vi "average_v2.vi"(4 "Numeric 8":fxp<+/-,24,1>, 5 "Numeric":fxp<+/-,24,1>, 6 "Numeric 7":fxp<+/-,24,1>, 7 "Numeric 2":fxp<+/-,24,1>, 8 "Numeric 6":fxp<+/-,24,1>, 9 "Numeric 5":fxp<+/-,24,1>, 10 "Numeric 4":fxp<+/-,24,1>, 11 "Numeric 3":fxp<+/-,24,1>) -> (1 "rms2":fxp<+/-,25,2> format="%.24g", 3 "mean":fxp<+/-,32,4>)   [LabVIEW 2014]
uses:
  <vilib>/rvi/Emulation/niFpgaProcessEmulError.vi
  <vilib>/rvi/FXPMathLib/FxpMul/XNode/nifxpmath_Multiplier.xnode
  <vilib>/rvi/FXPMathLib/FxpAdd/XNode/nifxpmath_Add.xnode
  <vilib>/rvi/FXPMathLib/sim/FxpSim.dll
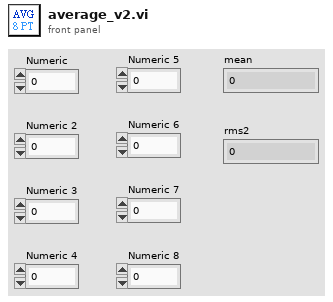
[diagram p1: front panel]
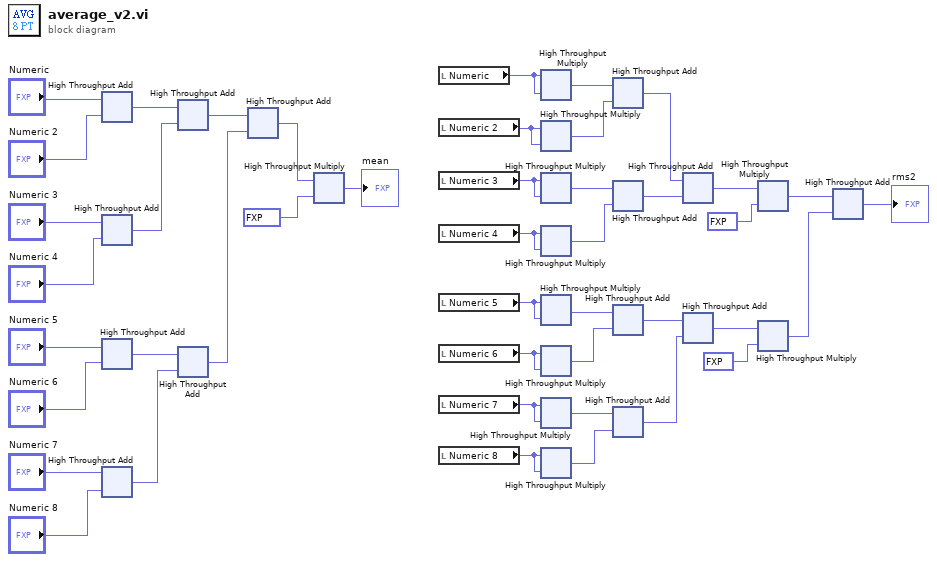
[diagram p0: block diagram]
diagram:
  n1 = xnode ("High Throughput Add")("x"="Numeric", "y"="Numeric 2") -> ("x+y"=w40:fxp<+/-,25,2>)
  n2 = xnode ("High Throughput Add")("x"="Numeric 3", "y"="Numeric 4") -> ("x+y"=w39:fxp<+/-,25,2>)
  n3 = xnode "High Throughput Add"("x"="Numeric 5", "y"="Numeric 6") -> ("x+y"=w20:fxp<+/-,25,2>)
  n4 = xnode "High Throughput Add"("x"="Numeric 7", "y"="Numeric 8") -> ("x+y"=w19:fxp<+/-,25,2>)
  n5 = xnode ("High Throughput Add")("x"=w40, "y"=w39) -> ("x+y"=w18:fxp<+/-,26,3>)
  n6 = xnode "High Throughput Add"("x"=w20, "y"=w19) -> ("x+y"=w17:fxp<+/-,26,3>)
  n7 = xnode "High Throughput Add"("x"=w18, "y"=w17) -> ("x+y"=w16:fxp<+/-,27,4>)
  n8 = xnode ("High Throughput Multiply")("x"=w16, "y"=fxp<+/-,5,0> 0.125) -> ("x*y"=→"mean":fxp<+/-,32,4>)
  n9 = local read "Numeric"() -> (w36:fxp<+/-,24,1>)
  n10 = local read "Numeric 2"() -> (w35:fxp<+/-,24,1>)
  n11 = local read "Numeric 3"() -> (w34:fxp<+/-,24,1>)
  n12 = local read "Numeric 4"() -> (w33:fxp<+/-,24,1>)
  n13 = local read "Numeric 5"() -> (w15:fxp<+/-,24,1>)
  n14 = local read "Numeric 6"() -> (w14:fxp<+/-,24,1>)
  n15 = local read "Numeric 7"() -> (w13:fxp<+/-,24,1>)
  n16 = local read "Numeric 8"() -> (w12:fxp<+/-,24,1>)
  n17 = xnode ("High Throughput Multiply")("x"=w36, "y"=w36) -> ("x*y"=w32:fxp<+/-,48,2>)
  n18 = xnode ("High Throughput Multiply")("x"=w35, "y"=w35) -> ("x*y"=w31:fxp<+/-,48,2>)
  n19 = xnode ("High Throughput Multiply")("x"=w34, "y"=w34) -> ("x*y"=w30:fxp<+/-,48,2>)
  n20 = xnode ("High Throughput Multiply")("x"=w33, "y"=w33) -> ("x*y"=w29:fxp<+/-,48,2>)
  n21 = xnode "High Throughput Multiply"("x"=w15, "y"=w15) -> ("x*y"=w11:fxp<+/-,48,2>)
  n22 = xnode "High Throughput Multiply"("x"=w14, "y"=w14) -> ("x*y"=w10:fxp<+/-,48,2>)
  n23 = xnode "High Throughput Multiply"("x"=w13, "y"=w13) -> ("x*y"=w9:fxp<+/-,48,2>)
  n24 = xnode "High Throughput Multiply"("x"=w12, "y"=w12) -> ("x*y"=w8:fxp<+/-,48,2>)
  n25 = xnode ("High Throughput Add")("x"=w32, "y"=w31) -> ("x+y"=w27:fxp<+/-,49,3>)
  n26 = xnode ("High Throughput Add")("x"=w30, "y"=w29) -> ("x+y"=w28:fxp<+/-,49,3>)
  n27 = xnode "High Throughput Add"("x"=w11, "y"=w10) -> ("x+y"=w7:fxp<+/-,49,3>)
  n28 = xnode "High Throughput Add"("x"=w9, "y"=w8) -> ("x+y"=w6:fxp<+/-,49,3>)
  n29 = xnode ("High Throughput Add")("x"=w27, "y"=w28) -> ("x+y"=w26:fxp<+/-,50,4>)
  n30 = xnode "High Throughput Add"("x"=w7, "y"=w6) -> ("x+y"=w4:fxp<+/-,50,4>)
  n31 = xnode ("High Throughput Multiply")("x"=w26, "y"=fxp<+/-,5,0> 0.25) -> ("x*y"=w3:fxp<+/-,24,1>)
  n32 = xnode ("High Throughput Multiply")("x"=w4, "y"=fxp<+/-,5,0> 0.25) -> ("x*y"=w2:fxp<+/-,24,1>)
  n33 = xnode "High Throughput Add"("x"=w3, "y"=w2) -> ("x+y"=→"rms2":fxp<+/-,25,2>)
